vi "MU Mt Analyze Result Optimal Spo_Mt.vi"(8 "error in (no error)":errorcluster, 11 "mtSyncAnalyzeResultHandle":T1) -> (0 "error out":errorcluster, 3 "optimalSpoMt":u8)   [LabVIEW 2017, in "MU_3SL_interface.lvlib"]
uses:
  MU_3SL_interface.lvlib
  handles/mtSyncAnalyzeResultHandle.ctl
  lib/MU_3SL_interface.dll
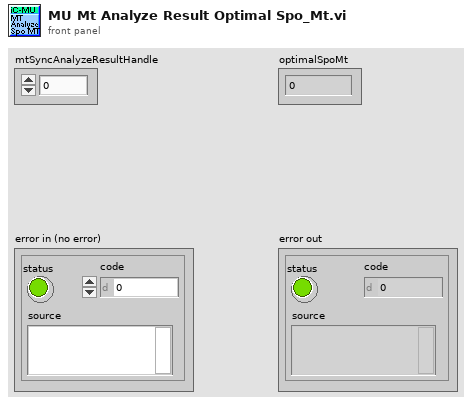
[diagram p1: front panel]
types:
  T1 = typedef "MU_3SL_interface.lvlib/mtSyncAnalyzeResultHandle.ctl" = u64
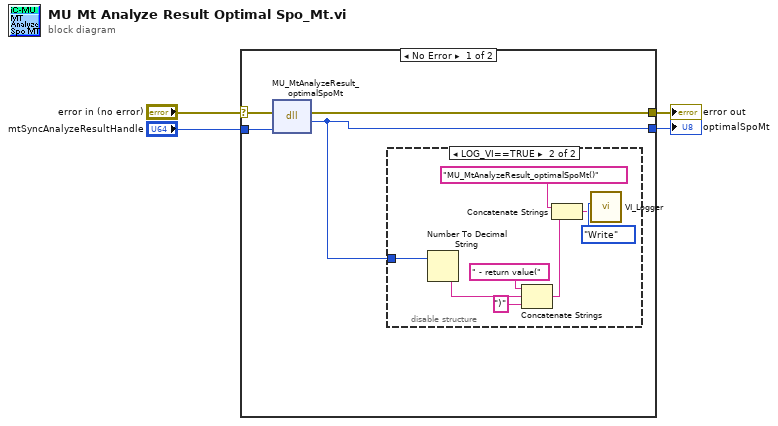
[diagram p0: block diagram]
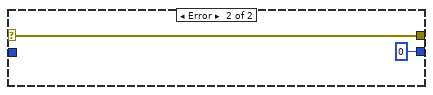
[diagram p3: hidden frame]
diagram:
  n1 = case shown="No Error" "error in (no error)" {
    selector: "error in (no error)" -> [w8 w18]
    tunnel: [w6 u8 0 ("optimalSpoMt")] -> w1
    tunnel: [w5 w18] -> w4
    tunnel: "mtSyncAnalyzeResultHandle" -> [w7 _]
    frame No Error {
      n2 = dll-call lib="C:/Users/bes/AppData/Roaming/work/mu_9so/icsubmodules/soft_mu_3sl_master/lv_interface/lib/MU_3SL_interface**.*" fn="MU_MtAnalyzeResult_optimalSpoMt"(error in=w8, "mtSyncAnalyzeResultHandle"=w7) -> (error out=w5:errorcluster, "optimalSpoMt"=w6:u8)  [unwired: 3 in, 1 out]
      n3 = disable-structure shown="LOG_VI==TRUE" {
        disable-tunnel: w6 -> [_ w10]
        frame condition #0 {
        }
        frame condition #1 (active) {
          n4 = Number To Decimal String(number=w10) -> (decimal integer string=w9:string)  [unwired: 1 in]
          n5 = Concatenate Strings(" - return value(" ("string"), w9, ")" ("string")) -> (w14:string)
          n6 = Concatenate Strings("MU_MtAnalyzeResult_optimalSpoMt()" ("Info in"), w14) -> (w13:string)
          n7 = call "VI_Logger.vi"("Action (Read)"=enum16{"Write", "Read"}."Write", "Info in"=w13) -> ()  [unwired: 8 in, 2 out]
        }
      }
    }
    frame Error {
    }
  }
  "error out" <- w4
  "optimalSpoMt" <- w1
